vi "sei_la.vi"(10 "INPUT":dbl) -> (2 "Output":dbl)   [LabVIEW 2020]
uses:
  GlobalVariables.vi
  <vilib>/Rock Robotics/Network Tables/NT Write Number.vi
panel:
  out "Disparo_Max":dbl
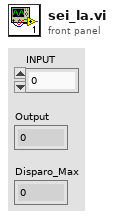
[diagram p1: front panel]
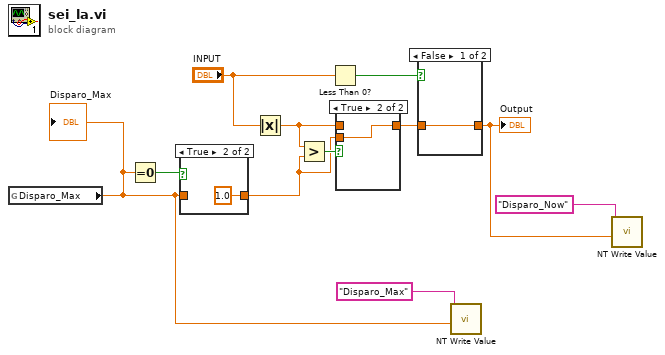
[diagram p0: block diagram]
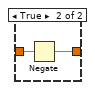
[diagram p3: hidden frame]
diagram:
  n1 = global read "GlobalVariables.vi" "Disparo_Max"() -> (w3:dbl)
  "Disparo_Max" <- w3
  n2 = Equal To 0?(x=w3) -> (x = 0?=w6:bool)
  n3 = case shown="True" w6 {
    tunnel: [w12 1.0 ("OVERRIDE")] -> w5
    tunnel: w3 -> [w12 _]
    frame False {
    }
    frame True {
    }
  }
  n4 = Absolute Value(x="INPUT") -> (abs(x)=w9:dbl)
  n5 = Greater?(x=w9, y=w5) -> (0:w11:bool)
  n6 = Less Than 0?(x="INPUT") -> (x < 0?=w8:bool)
  n7 = case shown="True" w11 {
    tunnel: [w14 w15] -> w7
    tunnel: w9 -> [w14 _]
    tunnel: w5 -> [_ w15]
    frame False {
    }
    frame True {
    }
  }
  n8 = case shown="False" w8 {
    tunnel: w7 -> [w16 w18]
    tunnel: [w16 w17] -> w1
    frame False {
    }
    frame True {
      n9 = Negate(x=w18) -> (-x=w17:dbl)
    }
  }
  "Output" <- w1
  n10 = call-poly <vilib>:"NT Write Value.vi"("Numeric"=w3, "Name"="Disparo_Max") -> ()  [unwired: 9 in, 1 out]
  n11 = call-poly <vilib>:"NT Write Value.vi"("Numeric"=w1, "Name"="Disparo_Now") -> ()  [unwired: 9 in, 1 out]
